vi "While Loop with Count Limit.vi"() -> ()   [LabVIEW 2016]
panel:
  out "Numeric 2":i32
  out "Numeric":i32
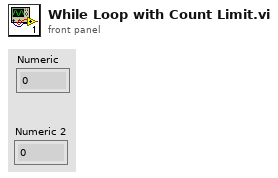
[diagram p1: front panel]
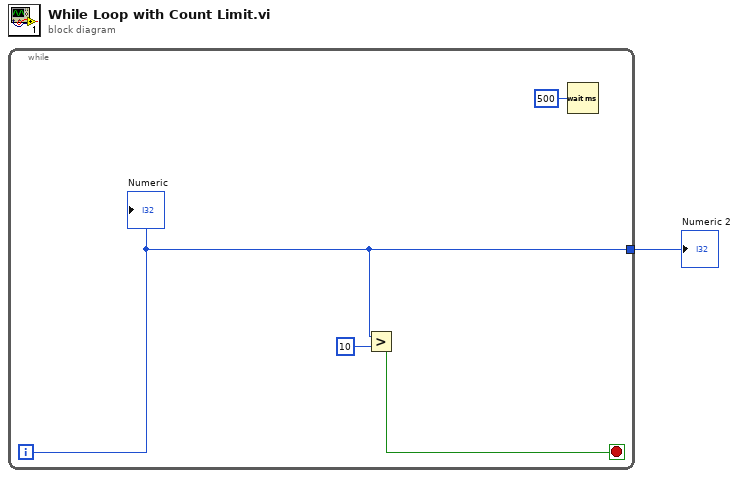
[diagram p0: block diagram]
diagram:
  n1 = while {
    tunnel: [w2] -> w1
    i -> [w2]
    stop <- w5 stop-if-true
    n2 = Greater?(x=w2, y=10) -> (0:w5:bool)
    n3 = Wait (ms)(milliseconds to wait=u32 500) -> ()  [unwired: 1 out]
    "Numeric" <- w2
  }
  "Numeric 2" <- w1
